vi "5-wire xVDT Sim.vi"(0 "Input Channel":refnum<k21>, 1 "Output Channels":cluster{"Out1":refnum<k21>, "Out2":refnum<k21>}, 2 "xVDT#.Scale1":fxp<+/-,19,5>, 3 "xVDT#.Scale2":fxp<+/-,19,5>, 4 "Last Value":i16) -> (5 "Next Value":i16)   [LabVIEW 2010]
uses:
  <vilib>/eio/EIONode/EIONode.xnode
  <vilib>/rvi/eio/nirviEIOImplementation/nirviEIOImplementation.xnode
  <vilib>/rvi/eio/common/nirviEmuClasses.ctl
  <vilib>/rvi/eio/common/nirviEmuTemplateMethod_noerrors.vi
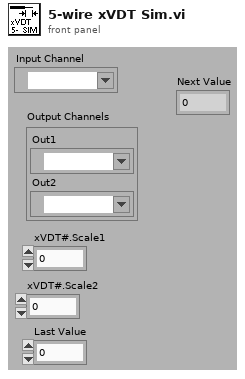
[diagram p1: front panel]
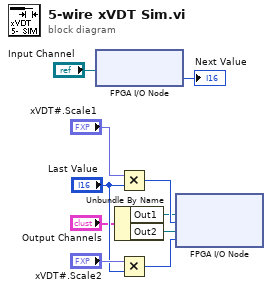
[diagram p0: block diagram]
diagram:
  n1 = xnode "FPGA I/O Node"("FPGA I/O In"="Input Channel") -> ("I/O Item"=→"Next Value":i16)  [unwired: 1 out]
  n2 = Unbundle By Name("Output Channels") -> ("Out1"=w2:refnum<k21>, "Out2"=w1:refnum<k21>)
  n3 = Multiply(x="xVDT#.Scale1", y="Last Value") -> (x*y=w7:i16)
  n4 = Multiply(x="xVDT#.Scale2", y="Last Value") -> (x*y=w4:i16)
  n5 = xnode "FPGA I/O Node"("I/O Item"=w7, "I/O Item"=w4, "FPGA I/O In"=w2, "FPGA I/O In"=w1) -> ()  [unwired: 2 out]
